vi "Run Pre-Render Hook.vi"(7 "Datum":refnum<class "Datum.lvclass">, 8 "Error In":errorcluster, 10 "Abstract Syntax Tree In":refnum<class "Root.lvclass">, 11 "Hooks In":T1) -> (0 "Error Out":errorcluster, 2 "Abstract Syntax Tree Out":refnum<class "Root.lvclass">, 3 "Hooks Out":T1)   [LabVIEW 2018, in "Toolkit.lvlib"]
uses:
  Data/Datum/Datum.lvclass
  Type Definitions/Hooks.ctl
  Hooks/Render/Render/Process.lvclass
  Hooks/Render/Section/Section.lvclass
  Hooks/Render/Variable/Variable.lvclass
  Nodes/Root/Root.lvclass
  Toolkit.lvlib
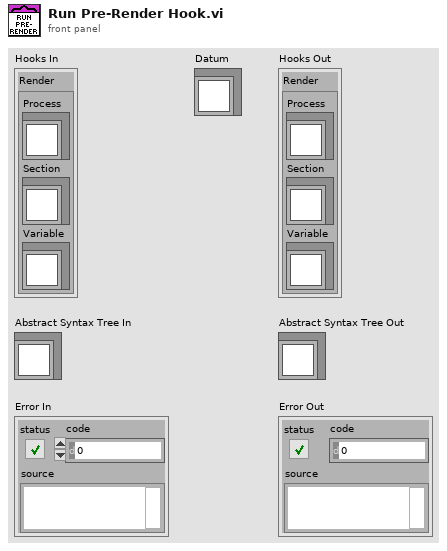
[diagram p1: front panel]
types:
  T1 = typedef "Toolkit.lvlib/Hooks.ctl" = cluster{"Render":cluster{"Process":refnum<class "Process.lvclass">, "Section":refnum<class "Section.lvclass">, "Variable":refnum<class "Variable.lvclass">}}
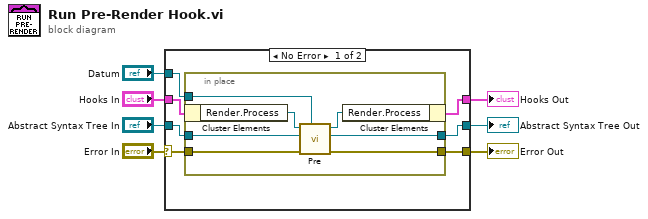
[diagram p0: block diagram]
diagram:
  n1 = case shown="No Error" "Error In" {
    selector: "Error In" -> [w8 w23]
    tunnel: "Datum" -> [w14 _]
    tunnel: [w13 w24] -> w6
    tunnel: "Hooks In" -> [w12 w24]
    tunnel: [w11 w22] -> w4
    tunnel: "Abstract Syntax Tree In" -> [w10 w22]
    tunnel: [w9 w23] -> w2
    frame No Error {
      n2 = in-place {
        in-place-border: w8 -> [w21]
        in-place-border: [w20] -> w9
        in-place-border: w10 -> [w19]
        in-place-border: [w18] -> w11
        in-place-border: w14 -> [w17]
        n3 = in-place-cluster #1(w12) -> ("Render.Process"=w16:refnum<class "Process.lvclass">)
        n4 = call-dynamic "Pre.vi"("Datum"=w17, "Error In"=w21, "Abstract Syntax Tree In"=w19, "Render In"=w16) -> ("Error Out"=w20:errorcluster, "Abstract Syntax Tree Out"=w18:refnum<class "Root.lvclass">, "Render Out"=w15:refnum<class "Process.lvclass">)  [unwired: 5 in]
        n5 = in-place-cluster #1("Render.Process"=w15) -> (w13:T1)
      }
    }
    frame Error {
    }
  }
  "Hooks Out" <- w6
  "Abstract Syntax Tree Out" <- w4
  "Error Out" <- w2
